vi "Main v1.2.vi"() -> ()   [LabVIEW 2017]
doc: "v0.85:\n- Counts for rejects and total\n\nv0.5:\n\n- Added Reject to Manual Mode\n- Send reject pallet cluster during manual mode\n- Run continuous manual happens only when no error has occured"
uses:
  Controls/Main Tabs v0.1.ctl
  Controls/Auto.ctl
  RT/Controls/Auto Delays.ctl
  RT/Controls/Auto Times.ctl
  support/Controls/General Para.ctl
  Controls/UI Data.ctl
  support/Controls/Auto Stats.ctl
  Controls/Logging FGV.ctl
  support/Message Queue/Enqueue Message (Single).vi
  GV/Maintenance GV.vi
  <vilib>/Utility/error.llb/Error Cluster From Error Code.vi
  <vilib>/ErrorRing/Error Ring.xnode
  support/Message Queue/Message Queue.lvlib
  support/User Event - Stop/User Event - Stop.lvlib
panel:
  in  "General Para 2":T1={"Max. Cons."=5.0, "Offset 1"=0.0, "Offset 2"=0.0, "Offset 3"=0.0, "Offset 4"=0.0} caption="General Para"
  in  "Auto Para 2":T2={"Agitator Delays"=[250, 350], "TF Delays"=[700, 800, 2], "Insertion Delays"=[100, 500], "Cutting Delays"=[300, 300, 100], "PF Delays"=[250, 30000], "Measur. Delays"=[500.0, 188.9, 1.0], "Reject Delays"=[500], "BF Delays"=[1000, 1000]}
  out "Shutdown?":bool
  out "Boolean 8":bool
  out "Boolean 7":bool
  out "Boolean 6":bool
  out "Boolean 5":bool
  out "Boolean 4":bool
  out "Boolean 3":bool
  out "Boolean 2":bool
  out "Boolean":bool
  in  "Reject Pallets":T3
  out "Date-Time":string caption="Dip-Tube Assembly Automation (HMI) v1.2"
  out "Main Tab":T4
  in  "All IOs":bool
  in  "Autocycle":T5
  in  "Manual":bool
  in  "Parameters":bool
  in  "Maintenance":bool
  in  "General Para":T1={"Max. Cons."=5.0, "Offset 1"=0.0, "Offset 2"=0.0, "Offset 3"=0.0, "Offset 4"=0.0} {"Offset 4" format="%.2f"; "Offset 3" format="%.2f"; "Offset 2" format="%.2f"; "Offset 1" format="%.2f"}
  in  "BF Para":cluster{"Delay 1":u32, "Delay 2":u32}={"Delay 1"=1000, "Delay 2"=1000}
  in  "Reject Para":cluster{"Delay":u32}={"Delay"=400}
  in  "Meas. Para":T6={"Delay"=500.0, "Mean Length"=188.9, "Tolerance"=1.0}
  in  "PF Para":cluster{"Delay":u32, "Timeout":u32}={"Delay"=1000, "Timeout"=1000}
  in  "Tube Feeder Para":T7={"Delay"=400, "Delay 2"=250, "Max Attempts"=250}
  in  "Cutting Para":T8={"Delay"=400, "Delay 2"=250, "Delay 3"=250}
  in  "Agitator Para":cluster{"Delay":u32, "Timeout":u32}={"Delay"=400, "Timeout"=250}
  in  "Insertion Para":cluster{"Delay 1":u32, "Delay 2":u32}={"Delay 1"=1000, "Delay 2"=1000}
  in  "Save Para":bool
  in  "Home Para":bool
  out "OEE":dbl format="%#.1f"
  out "QUA":dbl=100.0 min=0.0 max=100.0 step=0.1
  in  "Ideal Time":dbl=2.0 min=0.0 max=100.0 step=0.1
  in  "AVL":dbl=100.0 min=0.0 max=100.0 step=0.1
  out "Rejects 2":u32 caption="Rejects"
  in  "Reset MCount":bool
  in  "Enable BF?":bool
  in  "Enable Agitate?":bool
  in  "Enable Reject?":bool
  in  "Toggle Motor":bool
  in  "Continuous?":bool
  in  "Enable Measure?":bool
  in  "Enable Index?":bool
  in  "Enable PF?":bool
  in  "Manual Para":T2={"Agitator Delays"=[400, 250], "TF Delays"=[700, 800, 2], "Insertion Delays"=[100, 500], "Cutting Delays"=[300, 300, 100], "PF Delays"=[250, 30000], "Measur. Delays"=[500.0, 188.9, 1.0], "Reject Delays"=[500], "BF Delays"=[1000, 1000]}
  in  "Enable Cutting?":bool
  in  "Enable Insertion?":bool
  in  "Run Manual":bool
  in  "Enable TF?":bool
  in  "Home Manual":bool
  out "Status 2":T10
  out "Measurements":T11 {"Height 1" format="%#.2f"; "Height 2" format="%#.2f"; "Height 3" format="%#.2f"; "Height 4" format="%#.2f"}
  out "Output Count":u32 caption="Output\nCount"
  out "PRF":dbl=100.0 min=0.0 max=100.0 step=0.1
  in  "End Cycle":bool
  out "Statuses":string[][](table)
  in  "All IO":bool
  in  "Stats":bool
  in  "Home AC":bool
  out "Status":string
  out "Good":u32 format="%06.0f"
  out "Cycle Time":dbl format="%0.2f"
  out "Rejects":u32 format="%06.0f"
  out "Total Count 2":u32 caption="Total Count"
  out "Avg. Time":dbl caption="Avg. Cycle Time (s)" format="%#.3f"
  out "Output Chart":T12(graph)
  out "Reject Count":u32
  out "Good Count":u32
  out "Total Time":dbl caption="Effective Cycle Time (s)" format="%#.3f"
  out "Time Chart":T13(graph)
  out "OEE Chart":T14(graph)
  out "Timestamp":string caption="Date & Timestamp"
  out "Latest Measure.":T15 caption="Latest Measurements" {"Length 1 (mm)" format="%#.2f"}
  out "Auto Times":T9
  in  "Back Stats":bool
  out "OEE 2":T14 caption="Latest Measurements" {"AVL" format="%#.1f"; "PRF" format="%#.1f"; "QUA" format="%#.1f"; "OEE" format="%#.1f"}
  out "Measurement Chart":T16(graph)
  in  "Home IOs":bool
  in  "Back IO":bool
  out "IAS 4":dbl format="%#.3f"
  out "IAS 3":dbl format="%#.3f"
  out "IAS 2":dbl format="%#.3f"
  out "IAS 1":dbl format="%#.3f"
  out "DI 1":T17
  out "DI 2":T18
  out "DO 1":T19
  in  "Exit":bool
  in  "Shutdown":bool
  # "HARMONY VISION DIP-TUBE ASSEMBLY AUTOMATION"
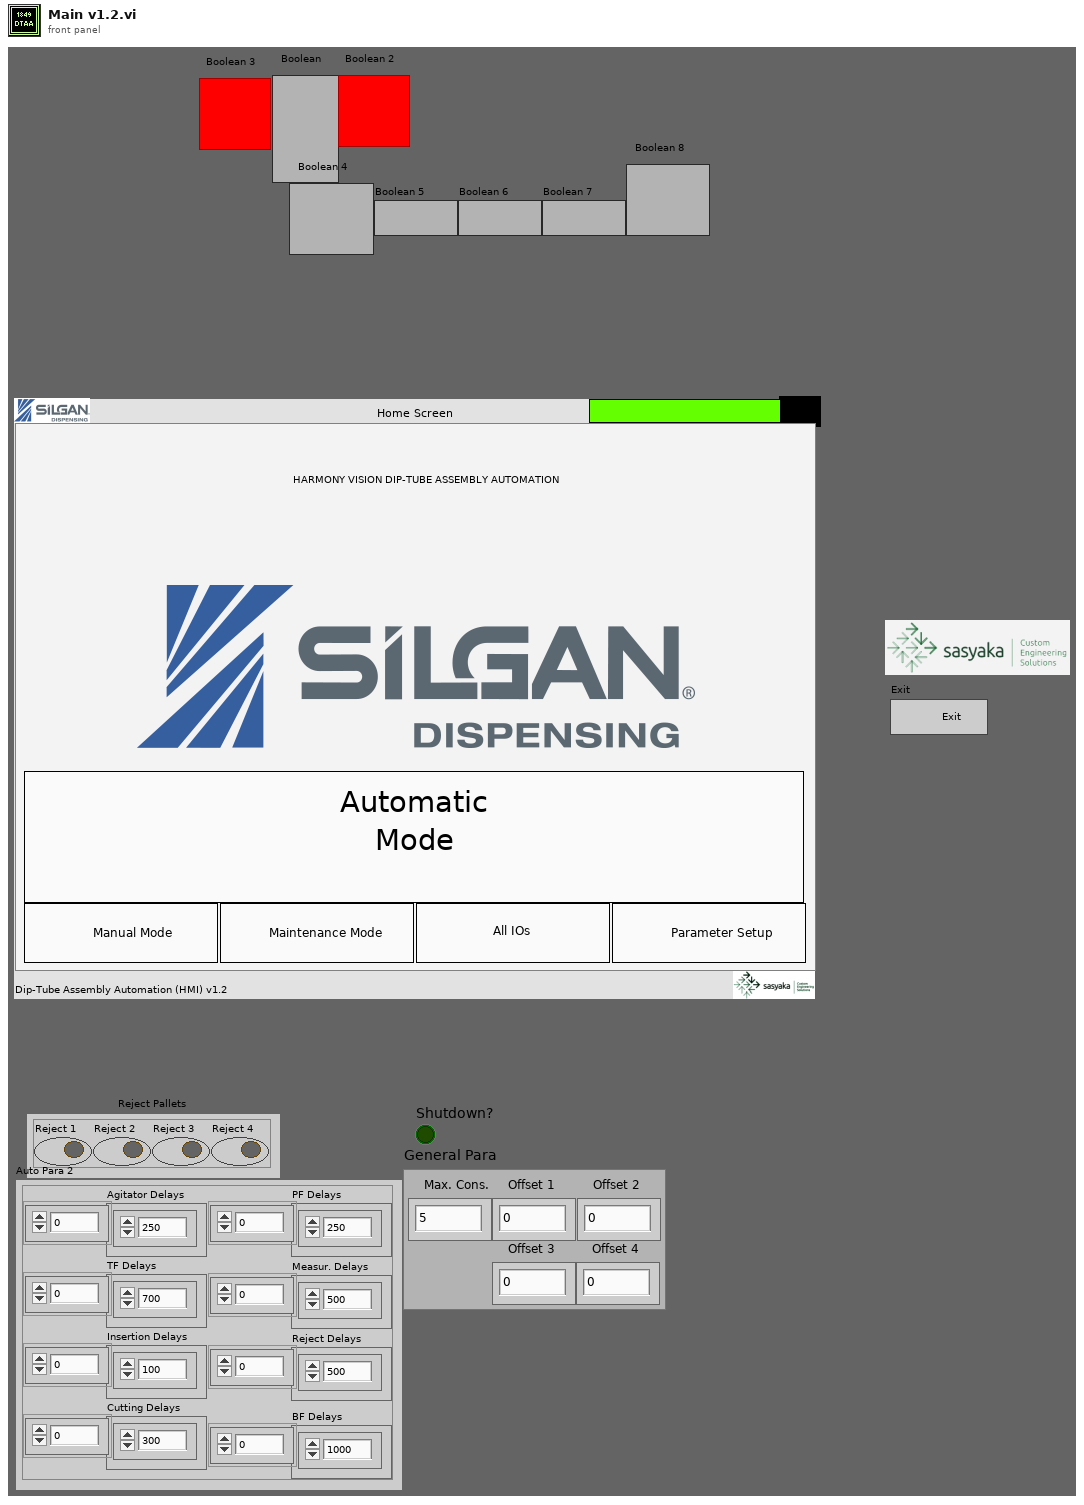
[diagram p1: front panel]
types:
  T1 = typedef "General Para.ctl" = cluster{"Max. Cons.":dbl, "Offset 1":dbl, "Offset 2":dbl, "Offset 3":dbl, "Offset 4":dbl}
  T2 = typedef "Auto Delays.ctl" = cluster{"Agitator Delays":u32[], "TF Delays":u32[], "Insertion Delays":u32[], "Cutting Delays":u32[], "PF Delays":u32[], "Measur. Delays":dbl[], "Reject Delays":u32[], "BF Delays":u32[]}
  T3 = cluster{"Reject 1":bool, "Reject 2":bool, "Reject 3":bool, "Reject 4":bool}
  T4 = typedef "Main Tabs v0.1.ctl" = enum32{"Home Screen", "Parameter Setup", "Manual Mode", "Autocycle", "Autocycle Statistics", "Autocycle IOs"}
  T5 = typedef "Auto.ctl" = bool
  T6 = cluster{"Delay":dbl, "Mean Length":dbl, "Tolerance":dbl}
  T7 = cluster{"Delay":u32, "Delay 2":u32, "Max Attempts":u32}
  T8 = cluster{"Delay":u32, "Delay 2":u32, "Delay 3":u32}
  T9 = typedef "Auto Times.ctl" = cluster{"Index Time":u32, "TF Time":u32, "Insertion Time":u32, "Cutting Time":u32, "PF Time":u32, "Meas. Time":u32, "Reject Time":u32}
  T10 = cluster{"Auto Times":T9, "error out":errorcluster}
  T11 = cluster{"Height 1":dbl, "Height 2":dbl, "Height 3":dbl, "Height 4":dbl}
  T12 = cluster{"OutputCount":u32, "Numeric Control":u32}
  T13 = cluster{"Index":dbl, "TF":dbl, "Insert":dbl, "Cutting":dbl, "PF":dbl, "Measure.":dbl, "Reject":dbl}
  T14 = cluster{"AVL":dbl, "PRF":dbl, "QUA":dbl, "OEE":dbl}
  T15 = cluster{"Length 1 (mm)":dbl, "Pallet 2 (mm)":dbl, "Pallet 3 (mm)":dbl, "Pallet 4 (mm)":dbl}
  T16 = cluster{"1":dbl, "2":dbl, "3":dbl, "4":dbl, "4":dbl, "4":dbl}
  T17 = cluster{"Machine_ON":bool, "E_stop ":bool, "SW_Pressure":bool, "SW_Start ":bool, "SW_Reset":bool, "SW_Stop":bool, "SW_Door":bool, "RS_Index_Rotary_CW":bool, "RS_Index_Rotary_CCW":bool, "RS_Index_Stopper _Rear":bool, "RS_Index_Output_Separator_Rear":bool, "PES_Index_Pallet_Sensor":bool, "PES_Index_Output_Part Sensor":bool, "ICS_BF_Low_Level_1":bool, "ICS_BF_Low_Level_2":bool, "ICS_BF_Pump_CNVR_Full_1":bool, "ICS_BF_Pump_CNVR_Full_2":bool, "ICS_BF_Pump_CNVR_Full_3":bool, "ICS_BF_Pump_CNVR_Full_4":bool, "PES_PC_Pump Presence_1":bool, "PES_PC_Pump Presence_2":bool, "PES_PC_Pump Presence_3":bool, "PES_PC_Pump Presence_4":bool, "RS_PC_Gating_Front":bool, "PES_Pump_Interference":bool, "PES_TF_Low_Level":bool, "PES_Tube Presence_1":bool, "PES_Tube Presence_2":bool, "PES_Tube Presence_3":bool, "PES_Tube Presence_4":bool, "DI1.30":bool, "DI1.31":bool}
  T18 = cluster{"RS_Agitatator_1_Rear ":bool, "RS_Agitatator_2_Rear ":bool, "RS_TF_Gating CYL_Rear":bool, "RS_Insertion_1_Rear":bool, "RS_Insertion_1_Front":bool, "RS_Insertion _2_Rear":bool, "RS_Insertion _2_Front":bool, "RS_Insertion _3_Rear":bool, "RS_Insertion _3_Front":bool, "RS_Insertion _4_Rear":bool, "RS_Insertion _4_Front":bool, "RS_Insertion_Clamp_Rear":bool, "RS_Cutting_Rear":bool, "RS_Cutting_Clamp _Rear":bool, "RS_Measurement_1_Rear":bool, "RS_Measurement_2_Rear":bool, "RS_Measurement_3_Rear":bool, "RS_Measurement_4_Rear":bool, "DI2.18":bool, "RS_Rejection_1_Rear":bool, "RS_Rejection_2_Rear":bool, "RS_Rejection_3_Rear":bool, "RS_Rejection_4_Rear":bool, "DI2.23":bool, "DI2.24":bool, "DI2.25":bool, "DI2.26":bool, "DI2.27":bool, "DI2.28":bool, "DI2.29":bool, "DI2.30":bool, "DI2.31":bool}
  T19 = cluster{"TL_Red":bool, "TL_Orange":bool, "TL_Green":bool, "TL_Buzzer":bool, "SOL_Index_Rotary_CW":bool, "SOL_Index_Rotary_CCW":bool, "SOL_Index_Stopper_Rear":bool, "SOL_OutputSeparator_Rear":bool, "Bowl  Feeder_ ON 1":bool, "Pump_CNVR_Motor _ON":bool, "SOL_PC_Gating_CYL_Rear":bool, "SOL_Tube_Feed_Agitatator":bool, "SOL_Tube_Feed_Gating_CYL":bool, "SOL_Insertion _CYL":bool, "SOL_Insertion_Clamp_CYL":bool, "SOL_Cutting_CYL":bool, "SOL_Cutting_Clamp_CYL":bool, "SOL_Insertion_Air_Nozzle":bool, "SOL_Measurement_CYL":bool, "DO1.19":bool, "SOL_Rejection CYL_1":bool, "SOL_Rejection CYL_2":bool, "SOL_Rejection CYL_3":bool, "SOL_Rejection CYL_4":bool, "Bowl  Feeder_ ON 2":bool, "SOL_BF_BlowerON":bool, "SOL_BF1_Track1":bool, "SOL_BF1_Track2":bool, "SOL_BF2_Track1":bool, "SOL_BF2_Track2":bool, "DO1.30":bool, "DO1.31":bool}
  T20 = typedef "UI Data.ctl" = cluster{"Main Tab":refnum<vi>}
  T21 = typedef "Message Queue.lvlib/All Message Queues.ctl" = cluster{"UI":refnum<queue>}
  T22 = enum8{"Enabled", "Disabled", "Disabled and Grayed Out"}
  T23 = cluster{"Array":string[][], "Machine Status":string}
  T24 = typedef "Logging FGV.ctl" = enum16{"Start Shift", "Log Index", "Read Shift", "Close Shift"}
  T25 = typedef "Auto Stats.ctl" = cluster{"Time-Stamp":timestamp, "Auto Times":T9, "Measurements":cluster{"1":dbl, "2":dbl, "3":dbl, "4":dbl}, "Outputs":cluster{"Good Parts":u32, "Reject Parts":u32}, "Cycle Time":dbl, "Remarks":string}
  T26 = cluster{"Auto Times":T9, "Results":cluster{"Measurements":cluster{"1":dbl, "2":dbl, "3":dbl, "4":dbl}, "Reject Pallets":cluster{"Reject 1":bool, "Reject 2":bool, "Reject 3":bool, "Reject 4":bool}}, "OutputCount":u32, "error out":errorcluster}
  T27 = enum8{"Information", "Error", "Successful", "Tips"}
  T28 = cluster{"Agitator Delays[0]":u32, "Agitator Delays[1]":u32}
  T29 = cluster{"TF Delays[0]":u32, "TF Delays[1]":u32, "TF Delays[2]":u32}
  T30 = cluster{"Insertion Delays[0]":u32, "Insertion Delays[1]":u32}
  T31 = cluster{"Cutting Delays[0]":u32, "Cutting Delays[1]":u32, "Cutting Delays[2]":u32}
  T32 = cluster{"Measur. Delays[0]":dbl, "Measur. Delays[1]":dbl, "Measur. Delays[2]":dbl}
  T33 = typedef "All Inputs.ctl" = cluster{"DI 1":cluster{"Machine_ON":bool, "E_stop ":bool, "SW_Pressure":bool, "SW_Start ":bool, "SW_Reset":bool, "SW_Stop":bool, "SW_Door":bool, "RS_Index_Rotary_CW":bool, "RS_Index_Rotary_CCW":bool, "RS_Index_Stopper _Rear":bool, "RS_Index_Output_Separator_Rear":bool, "PES_Index_Pallet_Sensor":bool, "PES_Index_Output_Part Sensor":bool, "ICS_BF_Low_Level_1":bool, "ICS_BF_Low_Level_2":bool, "ICS_BF_Pump_CNVR_Full_1":bool, "ICS_BF_Pump_CNVR_Full_2":bool, "ICS_BF_Pump_CNVR_Full_3":bool, "ICS_BF_Pump_CNVR_Full_4":bool, "PES_PC_Pump Presence_1":bool, "PES_PC_Pump Presence_2":bool, "PES_PC_Pump Presence_3":bool, "PES_PC_Pump Presence_4":bool, "RS_PC_Gating_Front":bool, "PES_Pump_Interference":bool, "PES_TF_Low_Level":bool, "PES_Tube Presence_1":bool, "PES_Tube Presence_2":bool, "PES_Tube Presence_3":bool, "PES_Tube Presence_4":bool, "DI1.30":bool, "DI1.31":bool}, "DI 2":cluster{"RS_Agitatator_1_Rear ":bool, "RS_Agitatator_2_Rear ":bool, "RS_TF_Gating CYL_Rear":bool, "RS_Insertion_1_Rear":bool, "RS_Insertion_1_Front":bool, "RS_Insertion _2_Rear":bool, "RS_Insertion _2_Front":bool, "RS_Insertion _3_Rear":bool, "RS_Insertion _3_Front":bool, "RS_Insertion _4_Rear":bool, "RS_Insertion _4_Front":bool, "RS_Insertion_Clamp_Rear":bool, "RS_Cutting_Rear":bool, "RS_Cutting_Clamp _Rear":bool, "RS_Measurement_1_Rear":bool, "RS_Measurement_2_Rear":bool, "RS_Measurement_3_Rear":bool, "RS_Measurement_4_Rear":bool, "RS_Measure_Clamp_Rear":bool, "RS_Rejection_1_Rear":bool, "RS_Rejection_2_Rear":bool, "RS_Rejection_3_Rear":bool, "RS_Rejection_4_Rear":bool, "DI2.23":bool, "DI2.24":bool, "DI2.25":bool, "DI2.26":bool, "DI2.27":bool, "DI2.28":bool, "DI2.29":bool, "DI2.30":bool, "DI2.31":bool}, "IAS 1":dbl, "IAS 2":dbl, "IAS 3":dbl, "IAS 4":dbl, "DO 1":cluster{"TL_Red":bool, "TL_Orange":bool, "TL_Green":bool, "TL_Buzzer":bool, "SOL_Index_Rotary_CW":bool, "SOL_Index_CNVR_Rotary_CCW":bool, "SOL_Index_CNVR_Stopper_Rear":bool, "SOL_Index_CNVR_Output _Separator _Rear":bool, "Bowl  Feeder_ ON 1":bool, "Pump_CNVR_Motor _ON":bool, "SOL_PC_Gating_CYL_Rear":bool, "SOL_Tube_Feed_Agitatator":bool, "SOL_Tube_Feed_Gating_CYL":bool, "SOL_Insertion _CYL":bool, "SOL_Insertion_Clamp_CYL":bool, "SOL_Cutting_CYL":bool, "SOL_Cutting_Clamp_CYL":bool, "SOL_Insertion_Air_Nozzle":bool, "SOL_Measurement_CYL":bool, "DO1.19":bool, "SOL_Rejection CYL_1":bool, "SOL_Rejection CYL_2":bool, "SOL_Rejection CYL_3":bool, "SOL_Rejection CYL_4":bool, "Bowl  Feeder_ ON 2":bool, "SOL_BF_BlowerON":bool, "SOL_BF1_Track1":bool, "SOL_BF1_Track2":bool, "SOL_BF2_Track1":bool, "SOL_BF2_Track2":bool, "DO1.30":bool, "DO1.31":bool}}
  T34 = cluster{"RS_Agitatator_1_Rear ":bool, "RS_Agitatator_2_Rear ":bool, "RS_TF_Gating CYL_Rear":bool, "RS_Insertion_1_Rear":bool, "RS_Insertion_1_Front":bool, "RS_Insertion _2_Rear":bool, "RS_Insertion _2_Front":bool, "RS_Insertion _3_Rear":bool, "RS_Insertion _3_Front":bool, "RS_Insertion _4_Rear":bool, "RS_Insertion _4_Front":bool, "RS_Insertion_Clamp_Rear":bool, "RS_Cutting_Rear":bool, "RS_Cutting_Clamp _Rear":bool, "RS_Measurement_1_Rear":bool, "RS_Measurement_2_Rear":bool, "RS_Measurement_3_Rear":bool, "RS_Measurement_4_Rear":bool, "RS_Measure_Clamp_Rear":bool, "RS_Rejection_1_Rear":bool, "RS_Rejection_2_Rear":bool, "RS_Rejection_3_Rear":bool, "RS_Rejection_4_Rear":bool, "DI2.23":bool, "DI2.24":bool, "DI2.25":bool, "DI2.26":bool, "DI2.27":bool, "DI2.28":bool, "DI2.29":bool, "DI2.30":bool, "DI2.31":bool}
  T35 = cluster{"TL_Red":bool, "TL_Orange":bool, "TL_Green":bool, "TL_Buzzer":bool, "SOL_Index_Rotary_CW":bool, "SOL_Index_CNVR_Rotary_CCW":bool, "SOL_Index_CNVR_Stopper_Rear":bool, "SOL_Index_CNVR_Output _Separator _Rear":bool, "Bowl  Feeder_ ON 1":bool, "Pump_CNVR_Motor _ON":bool, "SOL_PC_Gating_CYL_Rear":bool, "SOL_Tube_Feed_Agitatator":bool, "SOL_Tube_Feed_Gating_CYL":bool, "SOL_Insertion _CYL":bool, "SOL_Insertion_Clamp_CYL":bool, "SOL_Cutting_CYL":bool, "SOL_Cutting_Clamp_CYL":bool, "SOL_Insertion_Air_Nozzle":bool, "SOL_Measurement_CYL":bool, "DO1.19":bool, "SOL_Rejection CYL_1":bool, "SOL_Rejection CYL_2":bool, "SOL_Rejection CYL_3":bool, "SOL_Rejection CYL_4":bool, "Bowl  Feeder_ ON 2":bool, "SOL_BF_BlowerON":bool, "SOL_BF1_Track1":bool, "SOL_BF1_Track2":bool, "SOL_BF2_Track1":bool, "SOL_BF2_Track2":bool, "DO1.30":bool, "DO1.31":bool}
  T36 = cluster{"Manual Para":T2, "Reject Pallets":cluster{"Reject 1":bool, "Reject 2":bool, "Reject 3":bool, "Reject 4":bool}}
  T37 = cluster{"Measurements":cluster{"1":dbl, "2":dbl, "3":dbl, "4":dbl}, "Reject Pallets":cluster{"Reject 1":bool, "Reject 2":bool, "Reject 3":bool, "Reject 4":bool}}
  T38 = cluster{"Reject Pallets":cluster{"Reject 1":bool, "Reject 2":bool, "Reject 3":bool, "Reject 4":bool}, "Measurements":cluster{"1":dbl, "2":dbl, "3":dbl, "4":dbl}}
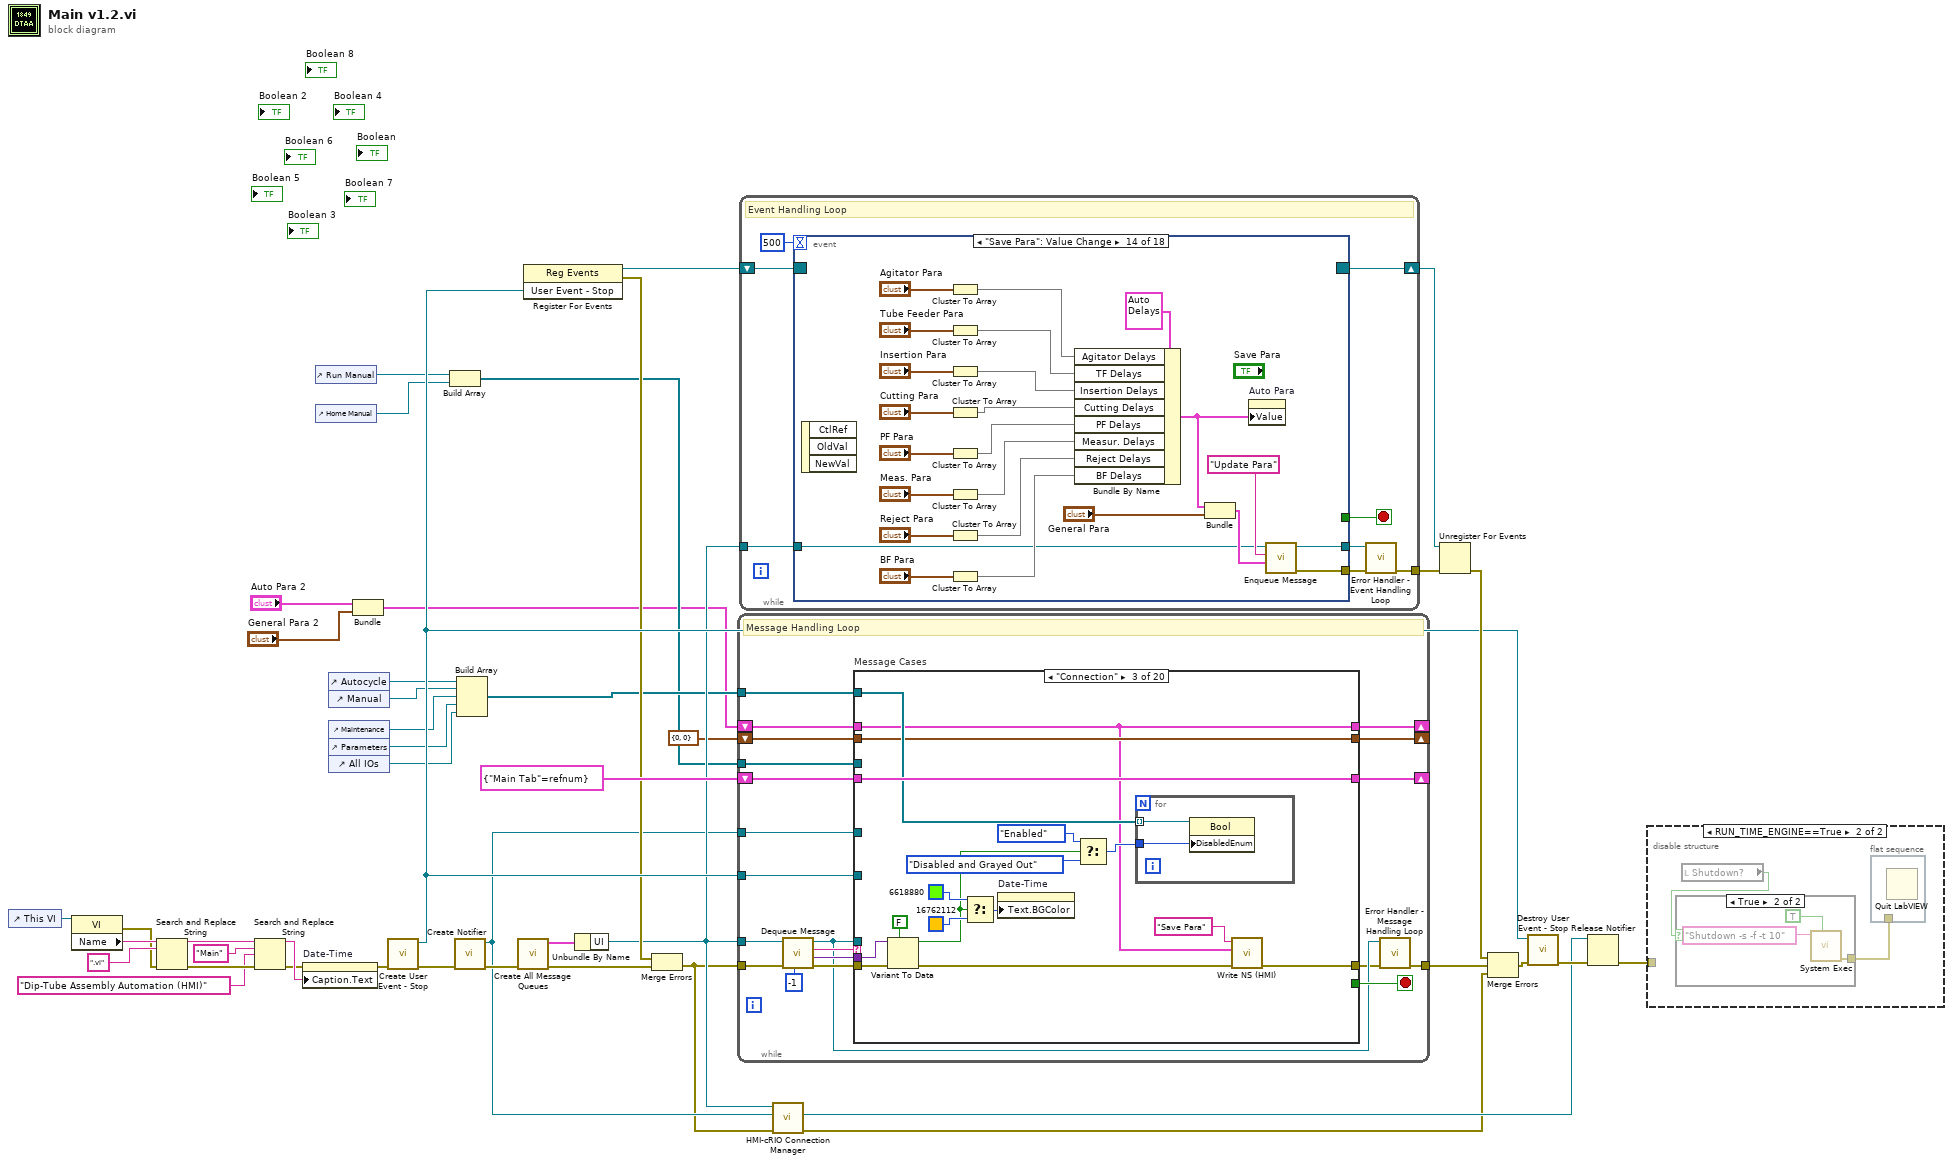
[diagram p0: block diagram]
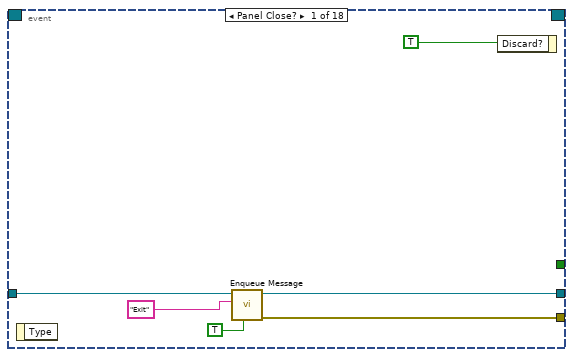
[diagram p2: hidden frame]
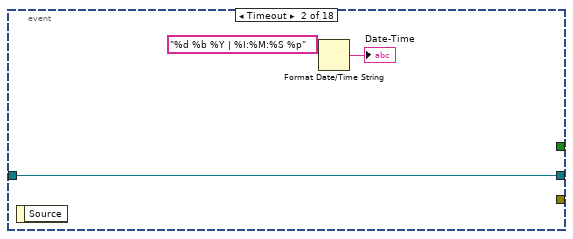
[diagram p3: hidden frame]
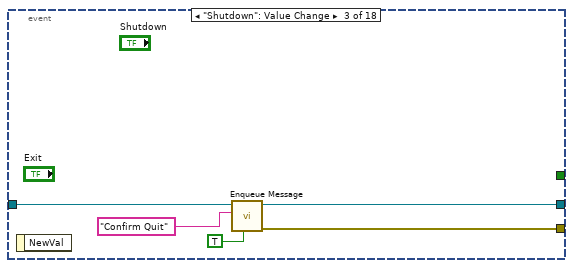
[diagram p4: hidden frame]
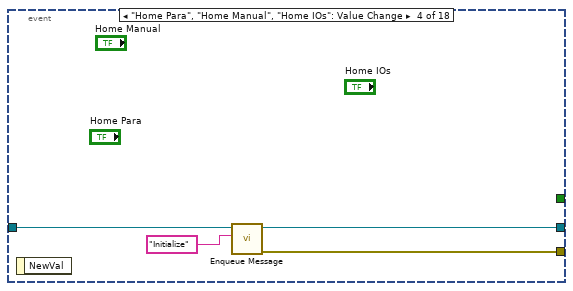
[diagram p5: hidden frame]
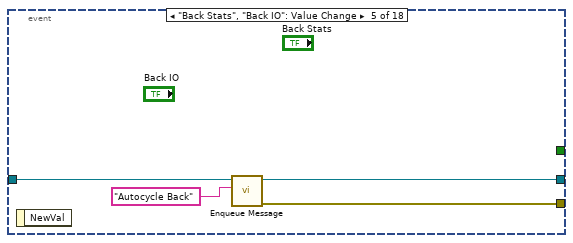
[diagram p6: hidden frame]
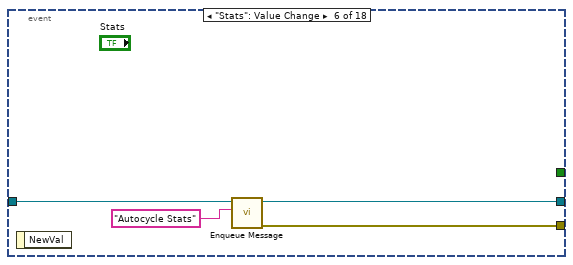
[diagram p7: hidden frame]
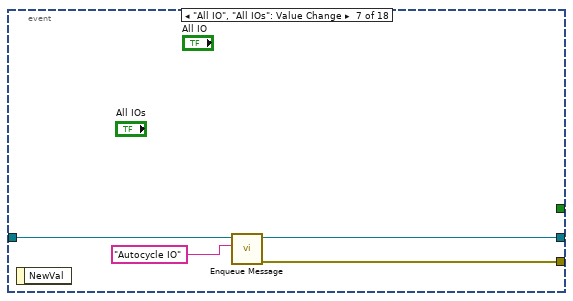
[diagram p8: hidden frame]
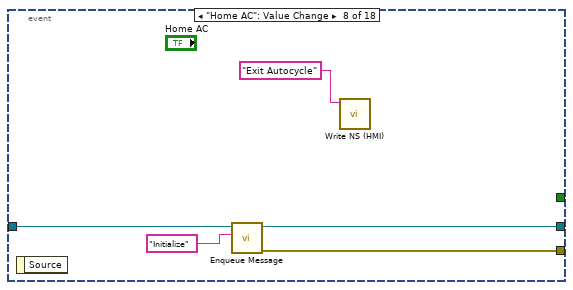
[diagram p9: hidden frame]
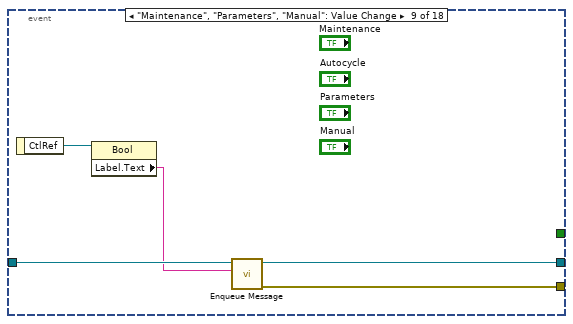
[diagram p10: hidden frame]
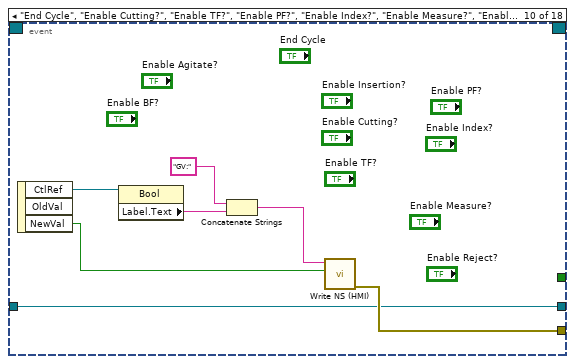
[diagram p11: hidden frame]
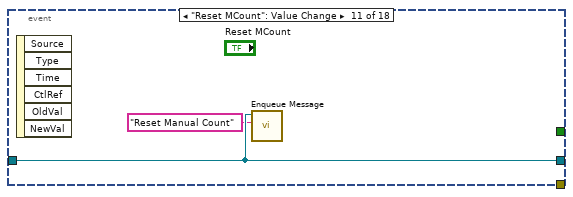
[diagram p12: hidden frame]
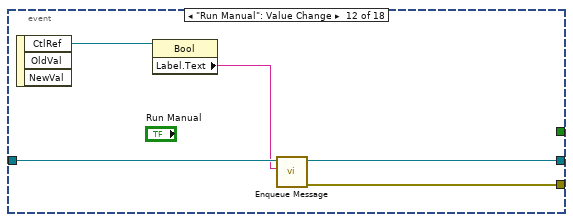
[diagram p13: hidden frame]
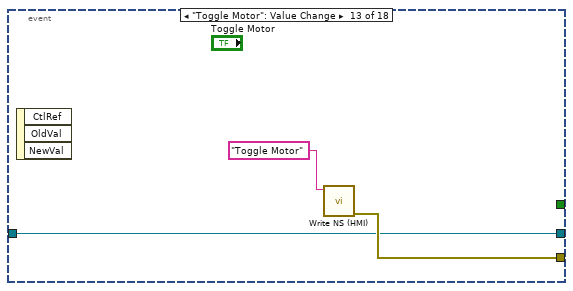
[diagram p14: hidden frame]
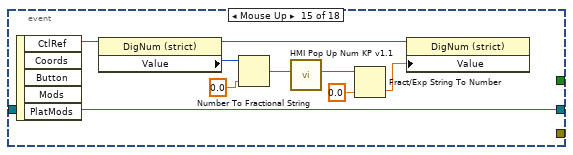
[diagram p15: hidden frame]
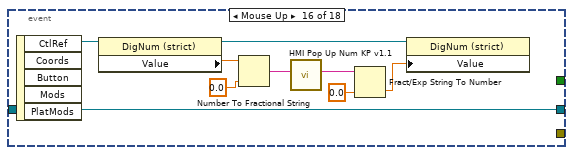
[diagram p16: hidden frame]
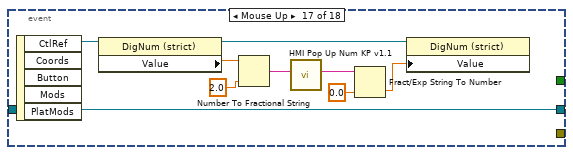
[diagram p17: hidden frame]
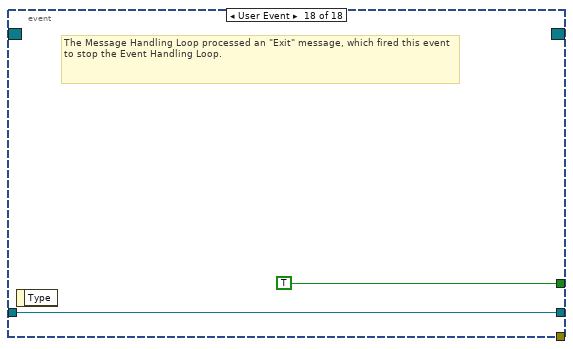
[diagram p18: hidden frame]
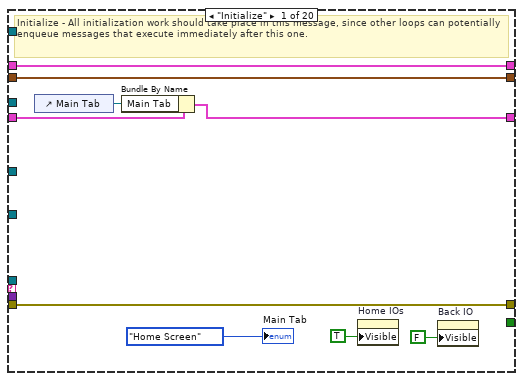
[diagram p19: hidden frame]
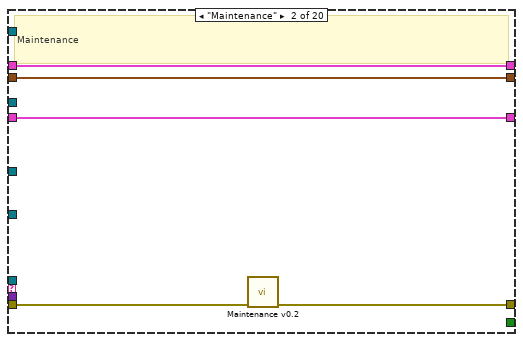
[diagram p20: hidden frame]
diagram:
  n1 = control-ref of="This VI"() -> (w15:refnum<vi>)
  n2 = property class="VI"(reference=w15) -> (error out=w14:errorcluster, "Name"=w21:string)  [unwired: 1 in, 1 out]
  n3 = Search and Replace String(input string=w21, search string=".vi", error in=w14) -> (result string=w19:string, error out=w18:errorcluster)  [unwired: 5 in, 2 out]
  n4 = Search and Replace String(input string=w19, search string="Main", replace string="Dip-Tube Assembly Automation (HMI)" ("replace string (\"\")"), error in=w18) -> (result string=w13:string, error out=w12:errorcluster)  [unwired: 4 in, 2 out]
  n5 = property on="Date-Time" class="Str"(error in=w12, "Caption.Text"=w13) -> (error out=w11:errorcluster)  [unwired: 1 in, 1 out]
  n6 = control-ref of="Run Manual"() -> (w10:refnum<vi>)
  n7 = control-ref of="Home Manual"() -> (w9:refnum<vi>)
  n8 = control-ref of="Autocycle"() -> (w26:refnum<vi>)
  n9 = control-ref of="Manual"() -> (w25:refnum<vi>)
  n10 = control-ref of="Maintenance"() -> (w24:refnum<vi>)
  n11 = control-ref of="Parameters"() -> (w23:refnum<vi>)
  n12 = control-ref of="All IOs"() -> (w4:refnum<vi>)
  n13 = Bundle("Auto Para 2"="Auto Para 2", "General Para 2"="General Para 2") -> (w1:cluster{"Auto Para 2":T2, "General Para 2":T1})  [unwired: 1 in]
  n14 = call "Create User Event - Stop.vi"("error in (no error)"=w11) -> ("error out"=w32:errorcluster, "User Event - Stop"=w35:refnum<user-event>)  [unwired: 9 in]
  n15 = Build Array(w10, w9) -> (w8:refnum<vi>[])
  n16 = call "Create Notifier.vi"("error in (no error)"=w32) -> ("error out"=w31:errorcluster, "notifier out"=w6:refnum<notifier>)  [unwired: 9 in]
  n17 = Build Array(w26, w25, w24, w23, w4) -> (w22:refnum<vi>[])
  n18 = call "Create All Message Queues.vi"("error in (no error)"=w31) -> ("error out"=w44:errorcluster, "Message Queues out"=w43:T21)  [unwired: 9 in]
  n19 = register-events(w35) -> (reference out=w36:refnum<event-registration>, error out=w34:errorcluster)  [unwired: 2 in]
  n20 = Unbundle By Name(w43) -> ("UI"=w33:refnum<queue>)
  n21 = Merge Errors(w34, w44) -> (w5:errorcluster)
  n22 = while {
    tunnel: w33 -> [w57]
    shift-right: [w64] -> _
    shift-left: T20 {"Main Tab"=refnum} ("Data Cluster") -> [w47]
    tunnel: w35 -> [w62]
    tunnel: w5 -> [w61]
    tunnel: [w55] -> w42
    tunnel: w6 -> [w52]
    tunnel: w22 -> [w51]
    tunnel: w8 -> [w50]
    shift-right: [w48] -> _
    shift-left: cluster{"OutputCount":u32, "RejectCount":u32} {"OutputCount"=0, "RejectCount"=0} -> [w49]
    shift-right: [w45] -> _
    shift-left: w1 -> [w46]
    stop <- w63 stop-if-true
    # "Message Handling Loop"
    n23 = call "Dequeue Message.vi"("timeout"=-1, "error in (no error)"=w61, "Message Queue"=w57) -> ("error out"=w60:errorcluster, "Message Data"=w58:variant, "Message"=w59:string, "dup Message Queue"=w56:refnum<queue>)  [unwired: 5 in]
    n24 = case "Message Cases" shown="\"Connection\"" w59 {
      selector: w59 -> [_ _ _ _ _ _ _ _ _ _ _ _ _ _ _ _ _ _ _ w375]
      tunnel: w56 -> [_ _ _ _ _ _ _ _ _ w181 w190 _ _ _ w294 _ _ w346 w372 _]
      tunnel: w60 -> [w73 w77 w93 w117 w128 w145 w153 w169 w175 w183 w198 w227 w258 w269 w302 w313 w337 w350 w365 _]
      tunnel: [w73 w76 w80 w117 w123 w145 w152 w169 w175 w182 w197 w228 w259 w271 w293 w313 w332 w348 w368 w376] -> w54
      tunnel: w47 -> [w72 w78 w95 w121 w130 w144 w149 w173 w179 w188 w195 w229 w260 w272 w303 w312 w336 w349 w371 w377]
      tunnel: [w71 w78 w95 w121 w130 w144 w149 w173 w179 w188 w195 w229 w260 w272 w303 w312 w336 w349 w371 w377] -> w64
      tunnel: [_ _ _ _ _ _ _ _ _ _ _ _ _ _ _ _ _ _ TRUE _] -> w63
      tunnel: w58 -> [_ _ w92 _ w127 _ _ _ _ _ _ w226 w257 _ w301 _ w335 _ w362 _]
      tunnel: w62 -> [_ _ _ _ _ _ _ _ _ _ _ _ _ _ _ _ _ _ w367 _]
      tunnel: w52 -> [_ _ _ _ _ _ _ _ _ _ _ _ _ _ _ _ _ _ w361 _]
      tunnel: w51 -> [_ _ w88 _ _ _ _ _ _ _ _ _ _ _ _ _ _ _ _ _]
      tunnel: w50 -> [_ _ _ _ _ _ _ _ _ _ _ _ _ w266 w299 _ _ _ _ _]
      tunnel: w49 -> [w68 w75 w83 w118 w129 w133 w154 w170 w176 w185 w199 w224 w255 w262 w292 _ w331 w345 w358 w374]
      tunnel: [w68 w75 w83 w118 w129 w133 w154 w170 w176 w185 w199 w224 w255 w262 w287 cluster{"OutputCount":u32, "RejectCount":u32} {"OutputCount"=0, "RejectCount"=0} w331 w345 w358 w374] -> w48
      tunnel: w46 -> [w65 w74 w79 w98 _ w132 w148 w168 w174 w180 w189 w213 w242 w261 w275 w309 w314 w338 w357 w373]
      tunnel: [w65 w74 w79 w98 w122 w132 w148 w168 w174 w180 w189 w213 w242 w261 w275 w309 w314 w338 w357 w373] -> w45
      frame "Initialize" {
        # "Initialize - All initialization work should take place in this message, since other loops can potentially enqueue messages that execute immediately after this one."
        n25 = control-ref of="Main Tab"() -> (w70:refnum<vi>)
        n26 = Bundle By Name(cluster=w72, "Main Tab"=w70) -> (w71:T20)
        n27 = property on="Home IOs" class="Bool"("Visible"=TRUE) -> ()  [unwired: 2 in, 2 out]
        n28 = property on="Back IO" class="Bool"("Visible"=FALSE) -> ()  [unwired: 2 in, 2 out]
        "Main Tab" <- Main_Tabs_v0.1."Home Screen" ("Main Tab")
      }
      frame "Maintenance" {
        # "Maintenance"
        n29 = call "Maintenance v0.2.vi"("Error In"=w77) -> ("Error out"=w76:errorcluster)  [unwired: 10 in]
      }
      frame "Connection" {
        n30 = Variant To Data(error in=w93, type=FALSE, Variant=w92) -> (data=w87:bool, error out=w81:errorcluster)
        n31 = Select(t=u32 6618880 ("Text.Text Colors:BG Color"), s=w87, f=u32 16762112 ("Text.Text Colors:BG Color")) -> (s? t:f=w89:u32)
        n32 = property on="Date-Time" class="Str"("Text.BGColor"=w89) -> ()  [unwired: 2 in, 2 out]
        n33 = Select(t=T22."Enabled" ("Disabled"), s=w87, f=T22."Disabled and Grayed Out") -> (s? t:f=w85:T22)
        n34 = for {
          tunnel: w88 -> [w97] mode=indexing
          tunnel: w85 -> [w96]
          n35 = property class="Bool"(reference=w97, "DisabledEnum"=w96) -> ()  [unwired: 1 in, 2 out]
        }
        n36 = call "Write NS (HMI).vi"("error in (no error)"=w81, "Message Data"=w79, "Message"="Save Para") -> ("error out"=w80:errorcluster)  [unwired: 8 in]
      }
      frame "Parameters" {
        # "Parameters"
        n37 = Unbundle(w98) -> ("Auto Para 2"=w100:T2, "General Para 2"=w99:T1)
        n38 = Unbundle By Name(w121) -> ("Main Tab"=w120:refnum<vi>)
        n39 = property on="General Para" class="Clust (strict)"("Value"=w99) -> ()  [unwired: 2 in, 2 out]
        n40 = Unbundle(w100) -> ("Agitator Delays"=w116:u32[], "TF Delays"=w115:u32[], "Insertion Delays"=w114:u32[], "Cutting Delays"=w113:u32[], "PF Delays"=w112:u32[], "Measur. Delays"=w111:dbl[], "Reject Delays"=w110:u32[], "BF Delays"=w109:u32[])
        n41 = property class="TabCtl"(reference=w120, "Value"=Main_Tabs_v0.1."Parameter Setup" ("Main Tab")) -> ()  [unwired: 1 in, 2 out]
        n42 = Array To Cluster(array=w116) -> (cluster=w108:T28)
        n43 = Array To Cluster(array=w115) -> (cluster=w107:T29)
        n44 = Array To Cluster(array=w114) -> (cluster=w106:T30)
        n45 = Array To Cluster(array=w113) -> (cluster=w105:T31)
        n46 = Array To Cluster(array=w112) -> (cluster=w104:cluster{"PF Delays[0]":u32, "PF Delays[1]":u32})
        n47 = Array To Cluster(array=w111) -> (cluster=w103:T32)
        n48 = Array To Cluster(array=w110) -> (cluster=w102:cluster{"Reject Delays[0]":u32})
        n49 = Array To Cluster(array=w109) -> (cluster=w101:cluster{"BF Delays[0]":u32, "BF Delays[1]":u32})
        n50 = property on="Agitator Para" class="Clust (strict)"("Value"=w108) -> ()  [unwired: 2 in, 2 out]
        n51 = property on="Tube Feeder Para" class="Clust (strict)"("Value"=w107) -> ()  [unwired: 2 in, 2 out]
        n52 = property on="Insertion Para" class="Clust (strict)"("Value"=w106) -> ()  [unwired: 2 in, 2 out]
        n53 = property on="Cutting Para" class="Clust (strict)"("Value"=w105) -> ()  [unwired: 2 in, 2 out]
        n54 = property on="PF Para" class="Clust (strict)"("Value"=w104) -> ()  [unwired: 2 in, 2 out]
        n55 = property on="Meas. Para" class="Clust (strict)"("Value"=w103) -> ()  [unwired: 2 in, 2 out]
        n56 = property on="Reject Para" class="Clust (strict)"("Value"=w102) -> ()  [unwired: 2 in, 2 out]
        n57 = property on="BF Para" class="Clust (strict)"("Value"=w101) -> ()  [unwired: 2 in, 2 out]
      }
      frame "Update Para" {
        # "Parameters"
        n58 = Variant To Data(error in=w128, type=cluster{"Auto Para":T2, "General Para":T1} {"Auto Para"={"Agitator Delays"=[], "TF Delays"=[], "Insertion Delays"=[], "Cutting Delays"=[], "PF Delays"=[], "Measur. Delays"=[], "Reject Delays"=[], "BF Delays"=[]}, "General Para"={"Max. Cons."=0.0, "Offset 1"=0.0, "Offset 2"=0.0, "Offset 3"=0.0, "Offset 4"=0.0}} ("cluster"), Variant=w127) -> (data=w122:cluster{"Auto Para":T2, "General Para":T1}, error out=w124:errorcluster)
        n59 = call "Write NS (HMI).vi"("error in (no error)"=w124, "Message Data"=w122, "Message"="Save Para") -> ("error out"=w123:errorcluster)  [unwired: 8 in]
      }
      frame "Manual" {
        # "Parameters"
        n60 = control-ref of="Enable Index?"() -> (w141:refnum<vi>)
        n61 = control-ref of="Enable PF?"() -> (w140:refnum<vi>)
        n62 = control-ref of="Enable Cutting?"() -> (w139:refnum<vi>)
        n63 = control-ref of="Enable Insertion?"() -> (w138:refnum<vi>)
        n64 = control-ref of="Enable TF?"() -> (w137:refnum<vi>)
        n65 = control-ref of="Enable Measure?"() -> (w135:refnum<vi>)
        n66 = Unbundle By Name(w132) -> ("Auto Para 2"=w131:T2)
        n67 = control-ref of="Enable Reject?"() -> (w134:refnum<vi>)
        n68 = Build Array(w141, w140, w139, w138, w137, w135, w134) -> (w136:refnum<vi>[])
        n69 = property on="Auto Para" class="Clust (strict)"("Value"=w131) -> ()  [unwired: 2 in, 2 out]
        n70 = for {
          tunnel: w136 -> [w147] mode=indexing
          n71 = property class="Bool (strict)"(reference=w147, "Val(Sgnl)"=FALSE ("Value (Signaling)")) -> ()  [unwired: 1 in, 2 out]
        }
        n72 = Unbundle By Name(w144) -> ("Main Tab"=w143:refnum<vi>)
        n73 = property class="TabCtl"(reference=w143, "Value"=Main_Tabs_v0.1."Manual Mode" ("Main Tab")) -> ()  [unwired: 1 in, 2 out]
      }
      frame "Autocycle" {
        # "Parameters"
        n74 = call "Select Model v0.1.vi"() -> ("Cancel out"=w150:bool, "Model out"=w151:string)  [unwired: 9 in, 1 out]
        n75 = case shown="False" w150 {
          tunnel: w153 -> [w158 w167]
          tunnel: [w165 w167] -> w152
          tunnel: w151 -> [w164 _]
          tunnel: w149 -> [w161 _]
          tunnel: w148 -> [w155 _]
          frame False {
            n76 = Unbundle By Name(w161) -> ("Main Tab"=w163:refnum<vi>)
            n77 = call "Write NS (HMI).vi"("error in (no error)"=w158, "Message Data"=w155, "Message"="Save Para") -> ("error out"=w157:errorcluster)  [unwired: 8 in]
            n78 = property class="TabCtl"(reference=w163, "Value"=Main_Tabs_v0.1."Autocycle" ("Main Tab")) -> ()  [unwired: 1 in, 2 out]
            n79 = call "Write NS (HMI).vi"("error in (no error)"=w157, "Message Data"=w164, "Message"="Autocycle") -> ("error out"=w165:errorcluster)  [unwired: 8 in]
            n80 = property on="Home IOs" class="Bool"("Visible"=FALSE) -> ()  [unwired: 2 in, 2 out]
            n81 = property on="Back IO" class="Bool"("Visible"=TRUE) -> ()  [unwired: 2 in, 2 out]
          }
          frame True {
          }
        }
      }
      frame "Autocycle Back" {
        # "Parameters"
        n82 = Unbundle By Name(w173) -> ("Main Tab"=w172:refnum<vi>)
        n83 = property class="TabCtl"(reference=w172, "Value"=Main_Tabs_v0.1."Autocycle" ("Main Tab")) -> ()  [unwired: 1 in, 2 out]
      }
      frame "Autocycle Stats" {
        # "Parameters"
        n84 = Unbundle By Name(w179) -> ("Main Tab"=w178:refnum<vi>)
        n85 = property class="TabCtl"(reference=w178, "Value"=Main_Tabs_v0.1."Autocycle Statistics" ("Main Tab")) -> ()  [unwired: 1 in, 2 out]
      }
      frame "Autocycle IO" {
        # "Parameters"
        n86 = Unbundle By Name(w188) -> ("Main Tab"=w187:refnum<vi>)
        n87 = property class="TabCtl"(reference=w187, "Value"=Main_Tabs_v0.1."Autocycle IOs" ("Main Tab")) -> ()  [unwired: 1 in, 2 out]
        n88 = call-poly "Enqueue Message.vi"("error in (no error)"=w183, "Message"="Update IO", "Message Queue"=w181) -> ("error out"=w182:errorcluster)  [unwired: 7 in, 1 out]
      }
      frame "Update IO" {
        n89 = Unbundle By Name(w195) -> ("Main Tab"=w196:refnum<vi>)
        n90 = Wait (ms)(milliseconds to wait=u32 200) -> ()  [unwired: 1 out]
        n91 = property class="TabCtl"(reference=w196) -> ("Value"=w194:variant)  [unwired: 1 in, 2 out]
        n92 = Variant To Data(type=Main_Tabs_v0.1."Autocycle IOs" ("Main Tab"), Variant=w194) -> (data=w191:T4)  [unwired: 1 in, 1 out]
        n93 = global read "Maintenance GV.vi" "All IO"() -> (w200:T33)
        n94 = case shown="\"Autocycle IOs\"" w191 {
          tunnel: w198 -> [w208 w211]
          tunnel: [w208 w210] -> w197
          tunnel: w190 -> [_ w209]
          frame Default {
          }
          frame "Autocycle IOs" {
            n95 = call-poly "Enqueue Message.vi"("error in (no error)"=w211, "Message"="Update IO", "Message Queue"=w209) -> ("error out"=w210:errorcluster)  [unwired: 7 in, 1 out]
          }
        }
        n96 = Unbundle(w200) -> ("DI 1"=→"DI 1":T17, "DI 2"=→"DI 2":T34, "IAS 1"=→"IAS 1":dbl, "IAS 2"=→"IAS 2":dbl, "IAS 3"=→"IAS 3":dbl, "IAS 4"=→"IAS 4":dbl, "DO 1"=→"DO 1":T35)
      }
      frame "Update UI" {
        # "Update Display - Convert the message data to a string to display in the Data Display indicator."
        n97 = Variant To Data(error in=w227, type=T23 {"Array"=[], "Machine Status"=""} ("Status Cluster"), Variant=w226) -> (data=w222:T23, error out=w225:errorcluster)
        n98 = Unbundle(w222) -> ("Array"=→"Statuses":string[][], "Machine Status"=w220:string)
        "Status" <- w220
        n99 = Search and Replace String(input string=w220, search string="Autocycle is Running") -> (number of replacements=w218:i32)  [unwired: 6 in, 3 out]
        n100 = Greater Than 0?(x=w218) -> (x > 0?=w216:bool)
        n101 = Select(t=T22."Disabled and Grayed Out" ("Disabled"), s=w216, f=T22."Enabled" ("Disabled")) -> (s? t:f=w215:T22)
        n102 = property on="Home AC" class="Bool"("DisabledEnum"=w215) -> ()  [unwired: 2 in, 2 out]
        n103 = Merge Errors(w225) -> (w228:errorcluster)
      }
      frame "Autocycle Log" {
        # "Update Display - Convert the message data to a string to display in the Data Display indicator."
        n104 = Variant To Data(error in=w258, type=T25 {"Time-Stamp"=timestamp(0 s since 1904-01-01), "Auto Times"={"Index Time"=0, "TF Time"=0, "Insertion Time"=0, "Cutting Time"=0, "PF Time"=0, "Meas. Time"=0, "Reject Time"=0}, "Measurements"={"1"=0.0, "2"=0.0, "3"=0.0, "4"=0.0}, "Outputs"={"Good Parts"=0, "Reject Parts"=0}, "Cycle Time"=0.0, "Remarks"=""} ("Auto Stats"), Variant=w257) -> (data=w253:T25, error out=w256:errorcluster)
        n105 = Unbundle By Name(w253) -> ("Time-Stamp"=w251:timestamp, "Measurements"=w241:cluster{"1":dbl, "2":dbl, "3":dbl, "4":dbl}, "Outputs"=→"Output Chart":cluster{"Good Parts":u32, "Reject Parts":u32}, "Auto Times"=→"Auto Times":T9)
        "Latest Measure." <- w241
        n106 = call "Stats Unbundle.vi"("State"=Logging_FGV."Log Index", "Auto Stats"=w253) -> ("Cycle Time"=→"Cycle Time" →"Total Time":dbl, "Counters"=w246:cluster{"GoodCount":u32, "RejectCount":u32}, "OEE Cluster"=→"OEE Chart" →"OEE 2":T14, "Avg. Cycle Time"=→"Avg. Time":dbl, "Total Times"=→"Time Chart":T13)  [unwired: 4 in, 1 out]
        n107 = Unbundle By Name(w246) -> ("GoodCount"=w230:u32, "RejectCount"=w231:u32)
        "Rejects" <- w231
        "Good" <- w230
        "Good Count" <- w230
        "Reject Count" <- w231
        n108 = Unbundle(w241) -> ("1"=w240:dbl, "2"=w239:dbl, "3"=w238:dbl, "4"=w237:dbl)
        n109 = Add(x=w230, y=w231) -> (x+y=→"Total Count 2":u32)
        n110 = Bundle("1"=w240, "2"=w239, "3"=w238, "4"=w237, "4"=187.9, "4"=189.9) -> (→"Measurement Chart":T16)  [unwired: 1 in]
        n111 = Format Date/Time String(time format string (%c)="%d-%m-%Y | %H:%M:%S%3u", seconds (now)=w251) -> (date/time string=→"Timestamp":string)  [unwired: 1 in]
        n112 = Merge Errors(w256) -> (w259:errorcluster)
      }
      frame "Run Manual" {
        # "Update Manual mode"
        n113 = Bundle("Manual Para"="Manual Para", "Reject Pallets"="Reject Pallets") -> (w263:T36)  [unwired: 1 in]
        n114 = for {
          tunnel: w266 -> [w274] mode=indexing
          tunnel: T22."Disabled and Grayed Out" ("Disabled") -> [w273]
          n115 = property class="Bool"(reference=w274, "DisabledEnum"=w273) -> ()  [unwired: 1 in, 2 out]
        }
        n116 = call "Write NS (HMI).vi"("error in (no error)"=w269, "Message Data"=w263, "Message"="Manual Run") -> ("error out"=w268:errorcluster)  [unwired: 8 in]
        n117 = Merge Errors(w268) -> (w271:errorcluster)
      }
      frame "Manual Status" {
        n118 = Variant To Data(error in=w302, type=T26 {"Auto Times"={"Index Time"=0, "TF Time"=0, "Insertion Time"=0, "Cutting Time"=0, "PF Time"=0, "Meas. Time"=0, "Reject Time"=0}, "Results"={"Measurements"={"1"=0.0, "2"=0.0, "3"=0.0, "4"=0.0}, "Reject Pallets"={"Reject 1"=FALSE, "Reject 2"=FALSE, "Reject 3"=FALSE, "Reject 4"=FALSE}}, "OutputCount"=0, "error out"={"status"=FALSE, "code"=0, "source"=""}} ("cluster"), Variant=w301) -> (data=w298:T26, error out=w293:errorcluster)
        n119 = Unbundle(w298) -> ("Auto Times"=w297:T9, "Results"=w289:T37, "OutputCount"=w288:u32, "error out"=w291:errorcluster)
        n120 = for {
          tunnel: w299 -> [w308] mode=indexing
          tunnel: T22."Enabled" ("Disabled") -> [w307]
          n121 = property class="Bool"(reference=w308, "DisabledEnum"=w307) -> ()  [unwired: 1 in, 2 out]
        }
        n122 = Unbundle(w289) -> ("Measurements"=w277:cluster{"1":dbl, "2":dbl, "3":dbl, "4":dbl}, "Reject Pallets"=w278:T3)
        "Measurements" <- w277
        n123 = Bundle("Auto Times"=w297, "error out"=w291) -> (→"Status 2":T10)  [unwired: 1 in]
        n124 = Bundle("Reject Pallets"=w278, "Measurements"=w277) -> (w276:T38)  [unwired: 1 in]
        n125 = call "Counts Update (manual).vi"("output cluster"=w276, "Desired Cycle Time (s)"="Ideal Time", "AVL"="AVL", "OutputCount"=w288, "Counts in"=w292) -> ("OEE"=w282:T14, "Counts out"=w287:cluster{"OutputCount":u32, "RejectCount":u32})  [unwired: 5 in]
        n126 = Unbundle(w282) -> ("PRF"=→"PRF":dbl, "QUA"=→"QUA":dbl, "OEE"=→"OEE":dbl)  [unwired: 1 out]
        n127 = Unbundle(w287) -> ("OutputCount"=→"Output Count":u32, "RejectCount"=→"Rejects 2":u32)
        n128 = case shown="True" "Continuous?" {
          tunnel: w294 -> [_ w306]
          tunnel: w291 -> [_ w305]
          frame False {
          }
          frame True {
            # "Run if continuous is TRUE & No Error"
            n129 = call-poly "Enqueue Message.vi"("error in (no error)"=w305, "Message"="Run Manual", "Message Queue"=w306) -> ()  [unwired: 7 in, 2 out]
          }
        }
      }
      frame "Reset Manual Count" {
        w310 = u32 0 ("Rejects")
        n130 = local write "Rejects 2"(w310) -> ()
        n131 = local write "Output Count"(w310) -> ()
      }
      frame "Error" {
        w318 = 128  # call and forget
        # "Run async so that this loop will continue to run"
        # "Error"
        n132 = Variant To Data(error in=w337, type=errorcluster {"status"=FALSE, "code"=0, "source"=""} ("error constant"), Variant=w335) -> (data=w330:errorcluster, error out=w333:errorcluster)
        n133 = Unbundle By Name(w330) -> ("source"=w329:string)
        n134 = vi-ref "NewDialog.vi"() -> (w325:refnum<vi>)
        n135 = property class="VI"(reference=w325) -> (error out=w327:errorcluster, "Name"=w326:string)  [unwired: 1 in, 1 out]
        n136 = Search and Replace String(input string=w329, search string="<err>") -> (result string=w317:string)  [unwired: 6 in, 3 out]
        n137 = Open VI Reference(type specifier VI Refnum (for type only)=refnum<vi> refnum, vi path=w326, options=w318, error in (no error)=w327) -> (vi reference=w320:refnum<vi>, error out=w321:errorcluster)  [unwired: 2 in]
        n138 = call-by-ref "Start Asynchronous Call"(reference=w320, error in=w321, "inIcon"=T27."Error", "inTitle"="ERROR", "inMessage"=w317) -> (reference out=w323:refnum<vi>, error out=w322:errorcluster)  [unwired: 6 in, 3 out]
        n139 = Close Reference(reference=w323, error in (no error)=w322) -> (error out=w324:errorcluster)
        n140 = call <vilib>:"Simple Error Handler.vi"("error in (no error)"=w324) -> ()  [unwired: 4 in, 5 out]
        n141 = Merge Errors(w333) -> (w332:errorcluster)
      }
      frame "Confirm Quit" {
        # "Confirm Quit - Message that can confirm whether or not the user wants to exit the application."
        n142 = call "NewDialog.vi"("inIcon"=T27."Information", "inTitle"="SHUTDOWN?", "inButton2Text"="Shutdown", "inButton1Text"="", "inMessage"="Are you sure you want to shutdown?") -> ("outButton2"=w339:bool)  [unwired: 4 in, 2 out]
        "Shutdown?" <- w339
        n143 = case shown="True" w339 {
          tunnel: w350 -> [w351 w356]
          tunnel: [w351 w355] -> w347
          tunnel: w346 -> [_ w354]
          frame False {
          }
          frame True {
            n144 = call-poly "Enqueue Message.vi"("Priority Message? (F)"=TRUE, "error in (no error)"=w356, "Message"="Exit", "Message Queue"=w354) -> ("error out"=w355:errorcluster)  [unwired: 6 in, 1 out]
          }
        }
        n145 = Merge Errors(w347) -> (w348:errorcluster)
      }
      frame "Exit" {
        # "Stop the VI"
        # "Release the message queue reference"
        # "Exit - Exit the application."
        n146 = Variant To Data(type=errorcluster {"status"=FALSE, "code"=0, "source"=""} ("error constant"), Variant=w362) -> (data=w363:errorcluster)  [unwired: 1 in, 1 out]
        n147 = call <vilib>:"Simple Error Handler.vi"("error in (no error)"=w363) -> ()  [unwired: 4 in, 5 out]
        n148 = Send Notification(notification=TRUE, notifier=w361) -> (error out=w359:errorcluster)  [unwired: 1 in, 1 out]
        n149 = call "Fire User Event - Stop.vi"("User Event - Stop"=w367) -> ("error out"=w366:errorcluster)  [unwired: 10 in]
        n150 = Release Queue(queue=w372, error in (no error)=w365) -> (error out=w369:errorcluster)  [unwired: 1 in, 2 out]
        n151 = Merge Errors(w359, w366, w369) -> (w368:errorcluster)
      }
      frame Default {
        # "'Default' case only runs if there is a message that isn't defined in any of the other cases.  Output a programming error."
        n152 = xnode "Error Ring"("parameter 0"=w375) -> ("error out"=w376:errorcluster)
      }
    }
    n153 = call "Error Handler - Message Handling Loop.vi"("error in (no error)"=w54, "Message Queue"=w56) -> ("dup error in"=w55:errorcluster)  [unwired: 8 in, 1 out]
  }
  n154 = while {
    tunnel: w33 -> [w392]
    shift-right: [w390] -> w39
    shift-left: w36 -> [w391]
    tunnel: [w386] -> w37
    stop <- w388 stop-if-true
    # "Event Handling Loop"
    n155 = event shown="[13] \"Save Para\": Value Change" {
      selector: w391 -> [_ _ _ _ _ _ _ _ _ _ _ _ _ _ _ _ _ _]
      dyn-events: [_ _ _ _ _ _ _ _ _ _ _ _ _ _ _ _ _ _] -> w390
      timeout: 500 -> [_ _ _ _ _ _ _ _ _ _ _ _ _ _ _ _ _ _]
      tunnel: [_ _ _ _ _ _ _ _ _ _ _ _ _ _ _ _ _ TRUE ("Discard?")] -> w388
      tunnel: w392 -> [w397 w401 w406 w410 w414 w418 w422 w427 w432 w437 w441 w446 w448 w451 w482 w491 w500 w502]
      tunnel: [w396 _ w405 w409 w413 w417 w421 w426 w431 w438 _ w444 w449 w454 _ _ _ _] -> w389
      tunnel: [w395 w401 w404 w408 w412 w416 w420 w425 w430 w437 w441 w445 w448 w450 w482 w491 w500 w502] -> w387
      event Panel Close? {
        n156 = event-data() -> ()  [unwired: 1 in, 1 out]
        n157 = call-poly "Enqueue Message.vi"("Priority Message? (F)"=TRUE, "Message"="Exit", "Message Queue"=w397) -> ("error out"=w396:errorcluster, "dup Message Queue"=w395:refnum<queue>)  [unwired: 7 in]
        n158 = event-data("Discard?"=TRUE) -> ()  [unwired: 1 in, 1 out]
      }
      event Timeout {
        n159 = event-data() -> ()  [unwired: 1 in, 1 out]
        n160 = Format Date/Time String(time format string (%c)="%d %b %Y | %I:%M:%S %p") -> (date/time string=→"Date-Time":string)  [unwired: 2 in]
      }
      event "Shutdown": Value Change {
        n161 = event-data() -> ()  [unwired: 1 in, 1 out]
        n162 = call-poly "Enqueue Message.vi"("Priority Message? (F)"=TRUE, "Message"="Confirm Quit", "Message Queue"=w406) -> ("error out"=w405:errorcluster, "dup Message Queue"=w404:refnum<queue>)  [unwired: 7 in]
      }
      event "Home Para", "Home Manual", "Home IOs": Value Change {
        n163 = event-data() -> ()  [unwired: 1 in, 1 out]
        n164 = call-poly "Enqueue Message.vi"("Message"="Initialize", "Message Queue"=w410) -> ("error out"=w409:errorcluster, "dup Message Queue"=w408:refnum<queue>)  [unwired: 8 in]
      }
      event "Back Stats", "Back IO": Value Change {
        n165 = event-data() -> ()  [unwired: 1 in, 1 out]
        n166 = call-poly "Enqueue Message.vi"("Message"="Autocycle Back", "Message Queue"=w414) -> ("error out"=w413:errorcluster, "dup Message Queue"=w412:refnum<queue>)  [unwired: 8 in]
      }
      event "Stats": Value Change {
        n167 = event-data() -> ()  [unwired: 1 in, 1 out]
        n168 = call-poly "Enqueue Message.vi"("Message"="Autocycle Stats", "Message Queue"=w418) -> ("error out"=w417:errorcluster, "dup Message Queue"=w416:refnum<queue>)  [unwired: 8 in]
      }
      event "All IO", "All IOs": Value Change {
        n169 = event-data() -> ()  [unwired: 1 in, 1 out]
        n170 = call-poly "Enqueue Message.vi"("Message"="Autocycle IO", "Message Queue"=w422) -> ("error out"=w421:errorcluster, "dup Message Queue"=w420:refnum<queue>)  [unwired: 8 in]
      }
      event "Home AC": Value Change {
        n171 = event-data() -> ()  [unwired: 1 in, 1 out]
        n172 = call-poly "Enqueue Message.vi"("Message"="Initialize", "Message Queue"=w427) -> ("error out"=w426:errorcluster, "dup Message Queue"=w425:refnum<queue>)  [unwired: 8 in]
        n173 = call "Write NS (HMI).vi"("Message"="Exit Autocycle") -> ()  [unwired: 10 in, 1 out]
      }
      event "Maintenance", "Parameters", "Manual": Value Change {
        n174 = event-data() -> ("CtlRef"=w429:refnum<vi>)  [unwired: 1 in]
        n175 = property class="Bool"(reference=w429) -> ("Label.Text"=w428:string)  [unwired: 1 in, 2 out]
        n176 = call-poly "Enqueue Message.vi"("Message"=w428, "Message Queue"=w432) -> ("error out"=w431:errorcluster, "dup Message Queue"=w430:refnum<queue>)  [unwired: 8 in]
      }
      event "End Cycle", "Enable Cutting?", "Enable TF?", "Enable PF?", "Enable Index?", "Enable Measure?", "Enable Reject?", "Enable Agitate?", "Enable BF?": Value Change {
        n177 = event-data() -> ("CtlRef"=w439:refnum<vi>, "NewVal"=w433:bool)  [unwired: 1 in, 1 out]
        n178 = property class="Bool"(reference=w439) -> ("Label.Text"=w436:string)  [unwired: 1 in, 2 out]
        n179 = Concatenate Strings("GV:" ("string"), w436) -> (w434:string)
        n180 = call "Write NS (HMI).vi"("Message Data"=w433, "Message"=w434) -> ("error out"=w438:errorcluster)  [unwired: 9 in]
      }
      event "Reset MCount": Value Change {
        n181 = event-data() -> ()  [unwired: 1 in, 6 out]
        n182 = call-poly "Enqueue Message.vi"("Message"="Reset Manual Count", "Message Queue"=w441) -> ()  [unwired: 8 in, 2 out]
      }
      event "Run Manual": Value Change {
        n183 = event-data() -> ("CtlRef"=w443:refnum<vi>)  [unwired: 1 in, 2 out]
        n184 = property class="Bool"(reference=w443) -> ("Label.Text"=w442:string)  [unwired: 1 in, 2 out]
        n185 = call-poly "Enqueue Message.vi"("Message"=w442, "Message Queue"=w446) -> ("error out"=w444:errorcluster, "dup Message Queue"=w445:refnum<queue>)  [unwired: 8 in]
      }
      event "Toggle Motor": Value Change {
        n186 = event-data() -> ()  [unwired: 1 in, 3 out]
        n187 = call "Write NS (HMI).vi"("Message"="Toggle Motor") -> ("error out"=w449:errorcluster)  [unwired: 10 in]
      }
      event "Save Para": Value Change {
        n188 = event-data() -> ()  [unwired: 1 in, 3 out]
        n189 = Cluster To Array(cluster="Agitator Para") -> (array=w471:u32[])
        n190 = Cluster To Array(cluster="Tube Feeder Para") -> (array=w469:u32[])
        n191 = Cluster To Array(cluster="Insertion Para") -> (array=w467:u32[])
        n192 = Cluster To Array(cluster="Cutting Para") -> (array=w465:u32[])
        n193 = Cluster To Array(cluster="PF Para") -> (array=w463:u32[])
        n194 = Cluster To Array(cluster="Meas. Para") -> (array=w461:dbl[])
        n195 = Cluster To Array(cluster="Reject Para") -> (array=w459:u32[])
        n196 = Cluster To Array(cluster="BF Para") -> (array=w457:u32[])
        n197 = Bundle By Name(cluster=T2 {"Agitator Delays"=[1000], "TF Delays"=[1000], "Insertion Delays"=[1000], "Cutting Delays"=[1000], "PF Delays"=[1000], "Measur. Delays"=[1000.0], "Reject Delays"=[1000], "BF Delays"=[1000]} ("Auto Para"), "Agitator Delays"=w471, "TF Delays"=w469, "Insertion Delays"=w467, "Cutting Delays"=w465, "PF Delays"=w463, "Measur. Delays"=w461, "Reject Delays"=w459, "BF Delays"=w457) -> (w456:T2)
        n198 = Bundle("Auto Para"=w456, "General Para"="General Para") -> (w453:cluster{"Auto Para":T2, "General Para":T1})  [unwired: 1 in]
        n199 = property on="Auto Para" class="Clust (strict)"("Value"=w456) -> ()  [unwired: 2 in, 2 out]
        n200 = call-poly "Enqueue Message.vi"("Message Data"=w453, "Message"="Update Para", "Message Queue"=w451) -> ("error out"=w454:errorcluster, "dup Message Queue"=w450:refnum<queue>)  [unwired: 7 in]
      }
      event "Insertion Para.Delay 1", "Insertion Para.Delay 2", "Agitator Para.Delay", "Agitator Para.Timeout", "Cutting Para.Delay", "Cutting Para.Delay 2", "Cutting Para.Delay 3", "Tube Feeder Para.Delay", "Tube Feeder Para.Delay 2", "Tube Feeder Para.Max Attempts", "PF Para.Delay", "PF Para.Timeout", "Reject Para.Delay", "BF Para.Delay 1", "BF Para.Delay 2": Mouse Up {
        n201 = event-data() -> ("CtlRef"=w474:refnum<vi>)  [unwired: 1 in, 4 out]
        n202 = property class="DigNum (strict)"(reference=w474) -> (reference out=w477:refnum<vi>, "Value"=w478:u32)  [unwired: 1 in, 1 out]
        n203 = Number To Fractional String(number=w478, precision (6)=0.0 ("width (-)")) -> (F-format string=w476:string)  [unwired: 2 in]
        n204 = call "HMI Pop Up Num KP v1.1.vi"("String In"=w476) -> ("String Out"=w475:string)  [unwired: 9 in, 1 out]
        n205 = Fract/Exp String To Number(string=w475, default (0 dbl)=0.0 ("default (0 I32)")) -> (number=w480:dbl)  [unwired: 2 in, 1 out]
        n206 = property class="DigNum (strict)"(reference=w477, "Value"=w480) -> ()  [unwired: 1 in, 2 out]
      }
      event "Meas. Para.Delay": Mouse Up {
        n207 = event-data() -> ("CtlRef"=w483:refnum<vi>)  [unwired: 1 in, 4 out]
        n208 = property class="DigNum (strict)"(reference=w483) -> (reference out=w486:refnum<vi>, "Value"=w487:dbl)  [unwired: 1 in, 1 out]
        n209 = Number To Fractional String(number=w487, precision (6)=0.0 ("width (-)")) -> (F-format string=w485:string)  [unwired: 2 in]
        n210 = call "HMI Pop Up Num KP v1.1.vi"("String In"=w485) -> ("String Out"=w484:string)  [unwired: 9 in, 1 out]
        n211 = Fract/Exp String To Number(string=w484, default (0 dbl)=0.0 ("default (0 I32)")) -> (number=w489:dbl)  [unwired: 2 in, 1 out]
        n212 = property class="DigNum (strict)"(reference=w486, "Value"=w489) -> ()  [unwired: 1 in, 2 out]
      }
      event "Meas. Para.Mean Length", "Meas. Para.Tolerance": Mouse Up {
        n213 = event-data() -> ("CtlRef"=w492:refnum<vi>)  [unwired: 1 in, 4 out]
        n214 = property class="DigNum (strict)"(reference=w492) -> (reference out=w495:refnum<vi>, "Value"=w496:dbl)  [unwired: 1 in, 1 out]
        n215 = Number To Fractional String(number=w496, precision (6)=2.0 ("width (-)")) -> (F-format string=w494:string)  [unwired: 2 in]
        n216 = call "HMI Pop Up Num KP v1.1.vi"("String In"=w494) -> ("String Out"=w493:string)  [unwired: 9 in, 1 out]
        n217 = Fract/Exp String To Number(string=w493, default (0 dbl)=0.0 ("default (0 I32)")) -> (number=w498:dbl)  [unwired: 2 in, 1 out]
        n218 = property class="DigNum (strict)"(reference=w495, "Value"=w498) -> ()  [unwired: 1 in, 2 out]
      }
      event User Event {
        # "The Message Handling Loop processed an \"Exit\" message, which fired this event to stop the Event Handling Loop."
        n219 = event-data() -> ()  [unwired: 1 in, 1 out]
      }
    }
    n220 = call "Error Handler - Event Handling Loop.vi"("error in (no error)"=w389, "Message Queue"=w387) -> ("dup error in"=w386:errorcluster)  [unwired: 8 in, 1 out]
  }
  n221 = call "HMI-cRIO Connection Manager.vi"("error in"=w5, "notifier in"=w6, "Queue in"=w33) -> ("error out"=w27:errorcluster, "Notifier out"=w28:refnum<notifier>)  [unwired: 7 in]
  n222 = Unregister For Events(event registration refnum=w39, error in=w37) -> (error out=w40:errorcluster)
  n223 = Merge Errors(w40, w42, w27) -> (w41:errorcluster)
  n224 = call "Destroy User Event - Stop.vi"("error in (no error)"=w41, "User Event - Stop"=w35) -> ("error out"=w30:errorcluster)  [unwired: 9 in]
  n225 = Release Notifier(notifier=w28, error in (no error)=w30) -> (error out=w29:errorcluster)  [unwired: 1 in, 2 out]
  n226 = disable-structure shown="RUN_TIME_ENGINE==True" {
    disable-tunnel: w29 -> [_ _]
    frame condition #0 (active) {
    }
    frame condition #1 {
      n227 = local read "Shutdown?"() -> (w503:bool)
      n228 = case shown="True" w503 {
        tunnel: [_ w505] -> w504
        frame False {
        }
        frame True {
          n229 = call <vilib>:"System Exec.vi"("wait until completion? (T)"=TRUE, "command line"="Shutdown -s -f -t 10") -> ("error out"=w505:errorcluster)  [unwired: 6 in, 3 out]
        }
      }
      n230 = flat-sequence {
        tunnel: w504 -> [_]
        frame #0 {
          n231 = Quit LabVIEW() -> ()  [unwired: 1 in]
        }
      }
    }
  }
